vi "Write Refresh Timeout (ms).vi"(8 "error in (no error)":errorcluster, 10 "Refresh Timeout (ms)":i32=100, 11 "Orca-Flash 4.0 V2 in":refnum<class "Orca-Flash 4.0 V2.lvclass">) -> (0 "error out":errorcluster, 3 "Orca-Flash 4.0 V2 out":refnum<class "Orca-Flash 4.0 V2.lvclass">)   [LabVIEW 2018]
uses:
  Orca-Flash 4.0 V2.lvclass
  C:/LVCUR/flash-gordon/Hardware/Camera/Camera.lvclass
  C:/LVCUR/flash-gordon/Hardware/Device/Device.lvclass
  C:/Program Files/National Instruments/LabVIEW 2018/vi.lib/ActorFramework/Actor/Actor.lvclass
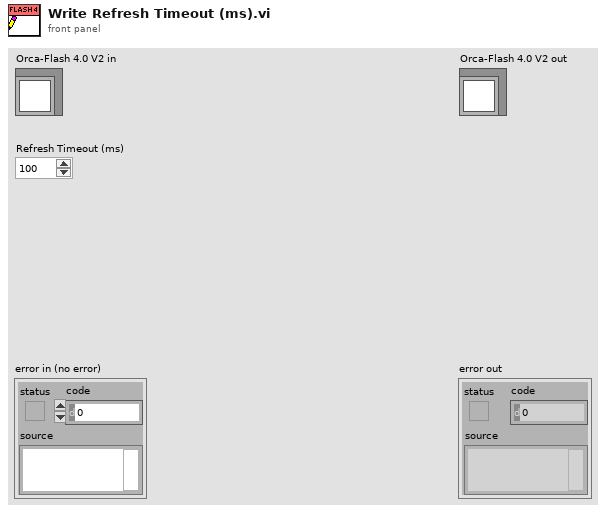
[diagram p1: front panel]
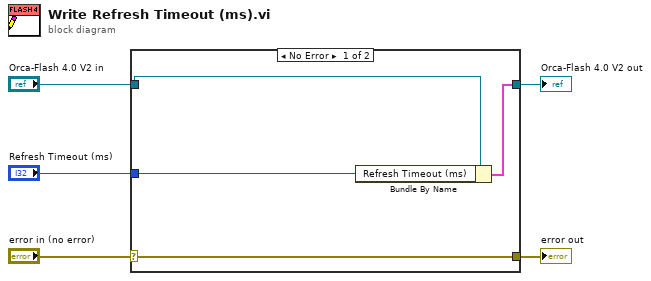
[diagram p0: block diagram]
diagram:
  n1 = case shown="No Error" "error in (no error)" {
    selector: "error in (no error)" -> [w9 w10]
    tunnel: [w9 w10] -> w4
    tunnel: [w7 w11] -> w2
    tunnel: "Orca-Flash 4.0 V2 in" -> [w8 w11]
    tunnel: "Refresh Timeout (ms)" -> [w6 _]
    frame No Error {
      n2 = Bundle By Name(cluster=w8, "Refresh Timeout (ms)"=w6) -> (w7:cluster{})
    }
    frame Error {
    }
  }
  "error out" <- w4
  "Orca-Flash 4.0 V2 out" <- w2
